vi "RT_stage_control_rev7.vi"() -> ()   [LabVIEW 2017]
uses:
  <vilib>/rvi/interface/nirviReadWriteControl/nirviReadWriteControl.xnode
  <vilib>/rvi/interface/nirviOpenFPGA/nirviOpenFPGA.xnode
  <vilib>/Platform/TimedLoop/XDataNode/XDataNode.xnode
  <vilib>/Platform/TimedLoop/XDataNode/nitl_modes.ctl
  <vilib>/Platform/TimedLoop/XDataNode/XDNodeRunTimeDep.lvlib
  <vilib>/Platform/TimedLoop/XDataNode/wakeup.ctl
  <vilib>/Platform/TimedLoop/XDataNode/timing_clust.ctl
  NiFpgaLv.dll
  <vilib>/Utility/error.llb/Error Cluster From Error Code.vi
  <vilib>/rvi/interface/Simulation/niFpgaSimulationCallBeginRW.vi
  <vilib>/rvi/errors/niLvFpgaAdjustHostInterfaceError.vi
  StageControl.ctl
  <vilib>/rvi/interface/nirviCloseFPGA/nirviCloseFPGA.xnode
  RasterControl.ctl
  <vilib>/FPGAPlugInAG/Dynamic/niLvFpga_Close_Dynamic.vi
  ForceControl.ctl
  FPGA Bitfiles/studentchallenge_FPGATarget_FPGARADCWDAC3_gNVwU-DQYMc.lvbitx
  FPGA_2R_ADC_W_DAC.vi
  <vilib>/FPGAPlugInAG/myRIO-1900/niLvFpga_Open_myRIO-1900.vi
  <vilib>/rvi/interface/common/dynamic/niFpgaDynamicAddResources.vi
panel:
  out "Force Loop":T1
  out "Force Control Late":i16
  in  "Y Manual [mm]":dbl format="%.4f"
  in  "X Manual [mm]":dbl format="%.4f"
  in  "Zero Cap":bool
  in  "Zero Y":bool
  in  "Zero X":bool
  in  "Des Force [N]":dbl=0.3 format="%.3f"
  in  "Return Speed":dbl=5.0 format="%#_13g"
  in  "Step Size [mm]":dbl=0.02 format="%.3f"
  in  "Width [mm]":dbl=3.0 format="%.3f"
  in  "Velocity [mm/s]":dbl=0.1 format="%.3f"
  in  "Stroke [mm]":dbl=3.0 format="%.3f"
  out "Current [A]":dbl=-0.00198361231060317 format="%.4f"
  out "Cap Probe [mm]":dbl=0.43435006179715263 format="%.4f"
  out "X Position [mm]":dbl format="%.4f"
  out "Y Position [mm]":dbl=0.0003125 format="%.4f"
  out "Stage Motion Late":i16
  in  "Start":bool
  in  "Operation":T2=enum."Raster"
  out "Raster Loop":T3
  out "Outer Loop":T2
  in  "stop":bool
  out "settle start":u32
  out "stroke finished":bool=TRUE
  out "ToolDownStart":bool
  out "Tool Up Finished":bool
  out "Tool Down Finished":bool
  out "FPGA Ref":refnum<k20>
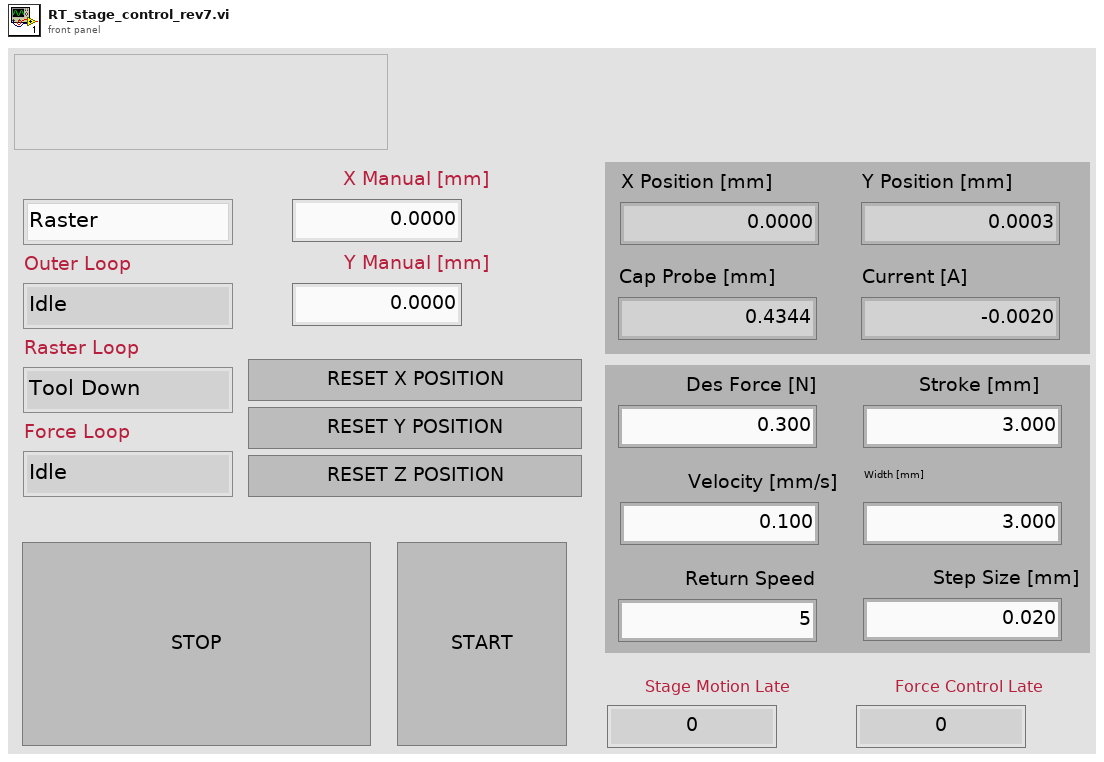
[diagram p1: front panel]
types:
  T1 = typedef "ForceControl.ctl" = enum16{"Idle", "Tool Down", "Force Control", "Tool Up"}
  T2 = typedef "StageControl.ctl" = enum16{"Idle", "Raster", "Home X", "Home Y"}
  T3 = typedef "RasterControl.ctl" = enum16{"Tool Down", "Stroke", "Tool Up", "Return & Step", "Settle", "Return to Zero"}
  T4 = cluster{"Encoder A":i32, "Encoder B":i32, "X Desired [mm]":dbl, "X Position [mm]":dbl, "Y Desired [mm]":dbl, "Y Position [mm]":dbl}
  T5 = typedef "XDNodeRunTimeDep.lvlib/timing_clust.ctl" = cluster{"Expected End [f-1]":u64, "Actual End [f-1]":u64, "Finished Late? [f-1]":bool, "Expected End [i-1]":u64, "Actual End [i-1]":u64, "Finished Late? [i-1]":bool, "Expected Start [i]":u64, "Actual Start [i]":u64, "Expected Start [f]":u64, "Actual Start [f]":u64, "Source Name":string, "Structure Name":string, "Period":i64, "Deadline":i64, "Offset":i64, "Start":i64, "Priority":i32, "Timeout":i32, "Mode":T6, "Wakeup Reason":T7, "Error":errorcluster, "Source Type":string, "Secondary Source Type":string, "Global End Time":u64, "Global Start Time":u64, "Frame Duration":u64, "Iteration Duration":u64, "Assigned CPU":i32, "I/O Scan Engine Mode":u32}
  T6 = typedef "XDNodeRunTimeDep.lvlib/nitl_modes.ctl" = enum32{"No Change", "Process missed periods, maintain original phase", "Discard missed periods, maintain original phase", "Process missed periods, ignore original phase", "Discard missed periods, ignore original phase"}
  T7 = typedef "XDNodeRunTimeDep.lvlib/wakeup.ctl" = enum32{"Normal", "Aborted", "Asynchronous wakeup", "Timing source error", "Timed loop error", "Timeout"}
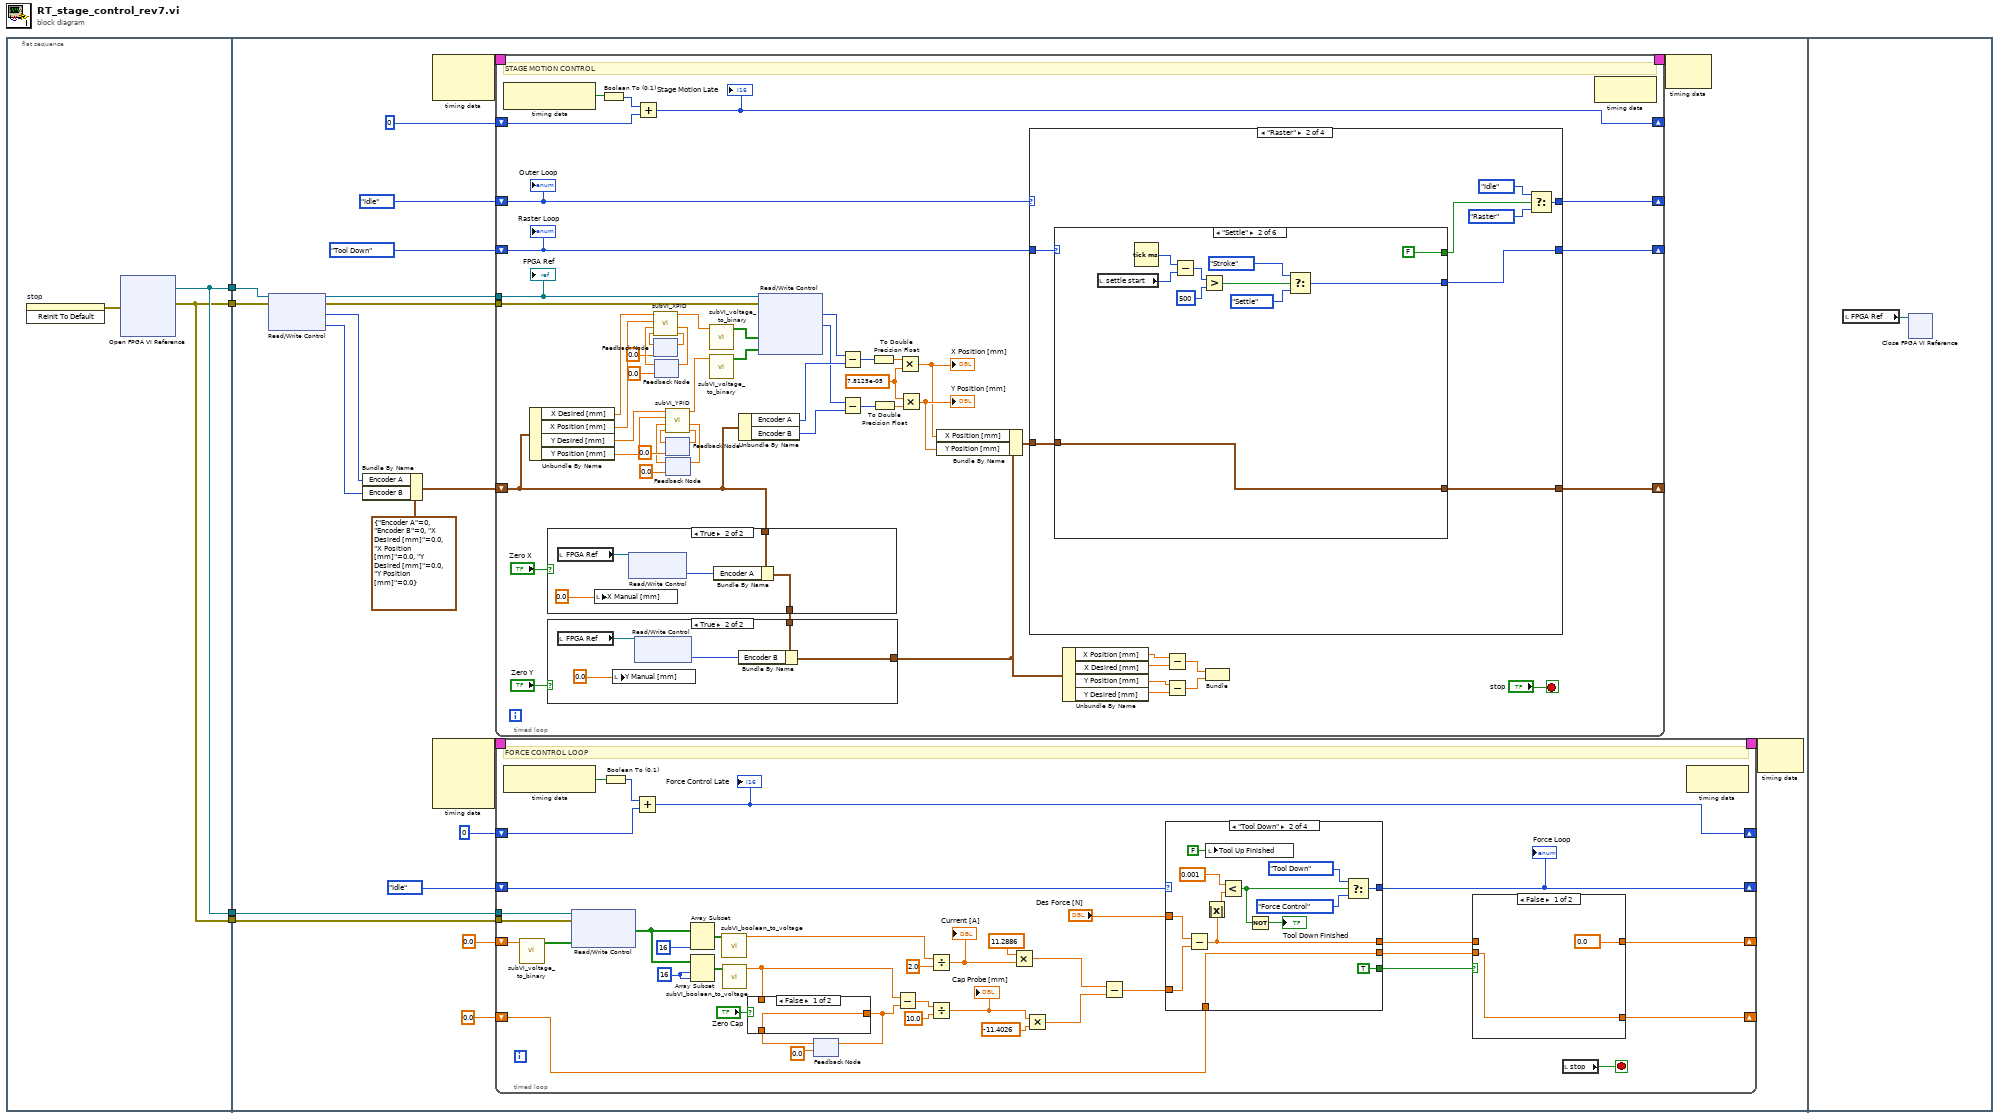
[diagram p0: block diagram]
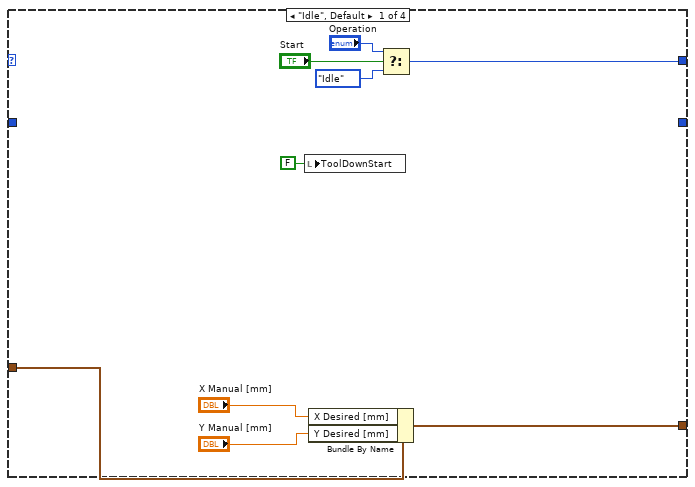
[diagram p2: hidden frame]
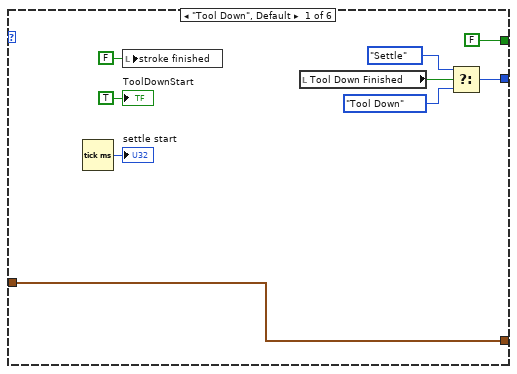
[diagram p3: hidden frame]
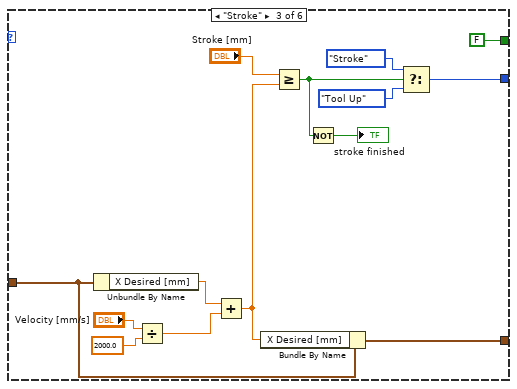
[diagram p4: hidden frame]
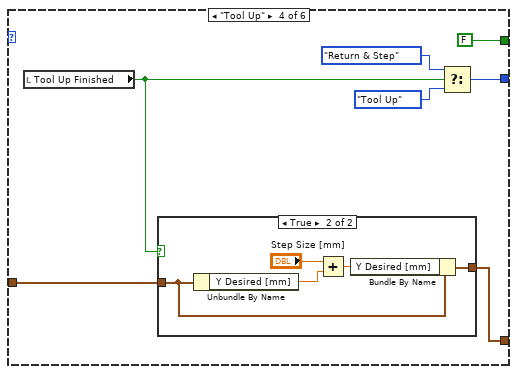
[diagram p5: hidden frame]
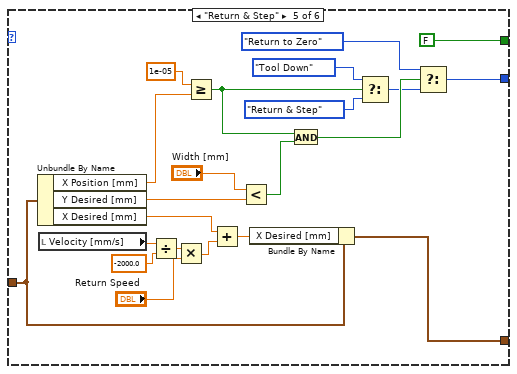
[diagram p7: hidden frame]
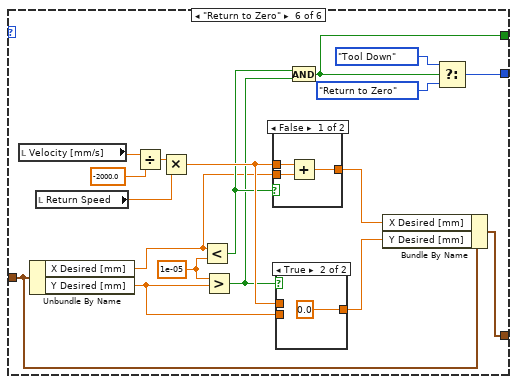
[diagram p8: hidden frame]
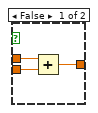
[diagram p9: hidden frame]
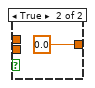
[diagram p10: hidden frame]
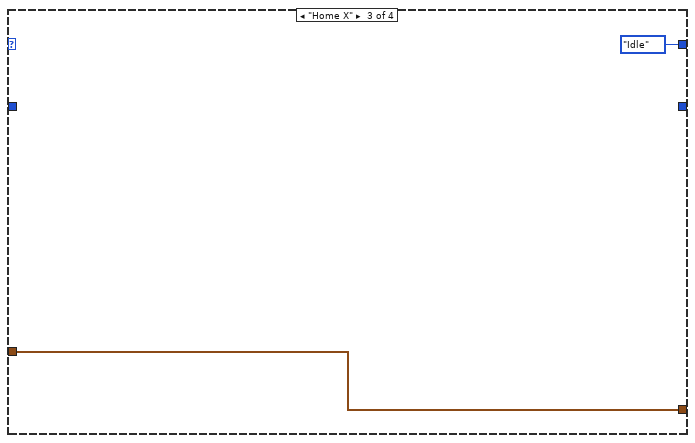
[diagram p11: hidden frame]
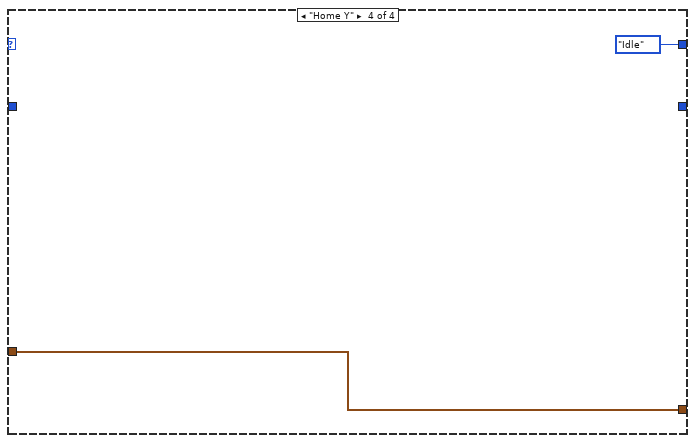
[diagram p12: hidden frame]
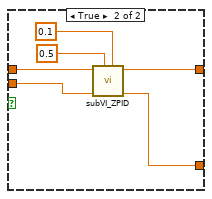
[diagram p15: hidden frame]
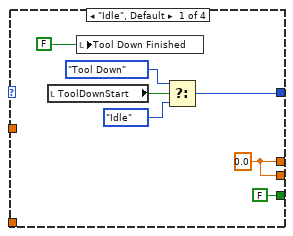
[diagram p17: hidden frame]
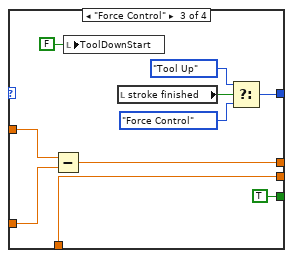
[diagram p18: hidden frame]
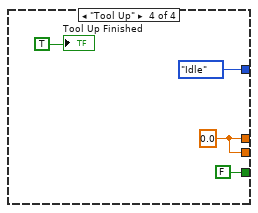
[diagram p19: hidden frame]
diagram:
  n1 = flat-sequence {
    tunnel: [w5] -> w4
    tunnel: [w6] -> w3
    tunnel: [w6] -> w2
    tunnel: [w5] -> w1
    tunnel: w4 -> [w19]
    tunnel: w3 -> [w17]
    tunnel: w2 -> [w16]
    tunnel: w1 -> [w15]
    frame #0 {
      n2 = invoke on="stop" class="Bool (strict)" method="Reinit To Default"() -> (error out=w7:errorcluster)  [unwired: 3 in, 2 out]
      n3 = xnode "Open FPGA VI Reference"("error in"=w7) -> ("FPGA VI Reference Out"=w6:refnum<k20>, "error out"=w5:errorcluster)  [unwired: 1 in]
    }
    frame #1 {
      n4 = xnode "Read/Write Control"("FPGA VI Reference In"=w17, "error in"=w19) -> ("FPGA VI Reference Out"=w24:refnum<k20>, "error out"=w23:errorcluster, "Encoder A"=w11:i32, "Encoder B"=w12:i32)
      n5 = Bundle By Name(cluster=T4 {"Encoder A"=0, "Encoder B"=0, "X Desired [mm]"=0.0, "X Position [mm]"=0.0, "Y Desired [mm]"=0.0, "Y Position [mm]"=0.0}, "Encoder A"=w11, "Encoder B"=w12) -> (w13:T4)
      n6 = node-c288() -> (w28:T5)  [unwired: 2 in]
      n7 = node-c288() -> (w26:T5)  [unwired: 4 in]
      n8 = timed-loop {
        timing: w28 -> [_]
        timing-out: [_] -> w27
        tunnel: w24 -> [w66]
        tunnel: w23 -> [w82]
        shift-right: [w76] -> _
        shift-left: StageControl."Idle" ("Enum 2") -> [w75]
        shift-right: [w73] -> _
        shift-left: RasterControl."Tool Down" -> [w74]
        shift-right: [w67] -> _
        shift-left: i16 0 -> [w68]
        shift-right: [w48] -> _
        shift-left: w13 -> [w43]
        stop <- "stop" stop-if-true
        w77 = 7.8125e-05 ("y")
        # "STAGE MOTION CONTROL"
        n9 = node-c288() -> (w70:bool)  [unwired: 1 in]
        n10 = Unbundle By Name(w43) -> ("X Desired [mm]"=w47:dbl, "X Position [mm]"=w46:dbl, "Y Desired [mm]"=w45:dbl, "Y Position [mm]"=w44:dbl)
        n11 = case shown="True" "Zero X" {
          tunnel: [w208 w210] -> w49
          tunnel: w43 -> [w208 w209]
          frame False {
          }
          frame True {
            n12 = local read "FPGA Ref"() -> (w212:refnum<k20>)
            n13 = local write "X Manual [mm]"(0.0 ("X Relative Position [mm]")) -> ()
            n14 = xnode "Read/Write Control"("FPGA VI Reference In"=w212) -> ("Encoder A"=w211:i32)  [unwired: 1 in, 2 out]
            n15 = Bundle By Name(cluster=w209, "Encoder A"=w211) -> (w210:T4)
          }
        }
        n16 = case shown="True" "Zero Y" {
          tunnel: w49 -> [w202 w206]
          tunnel: [w202 w203] -> w29
          frame False {
          }
          frame True {
            n17 = local read "FPGA Ref"() -> (w207:refnum<k20>)
            n18 = local write "Y Manual [mm]"(0.0 ("Y Relative Position [mm]")) -> ()
            n19 = xnode "Read/Write Control"("FPGA VI Reference In"=w207) -> ("Encoder B"=w205:i32)  [unwired: 1 in, 2 out]
            n20 = Bundle By Name(cluster=w206, "Encoder B"=w205) -> (w203:T4)
          }
        }
        n21 = Boolean To (0,1)(Boolean=w70) -> (0, 1=w69:i16)
        n22 = Add(x=w69, y=w68) -> (x+y=w67:i16)
        "Stage Motion Late" <- w67
        n23 = feedback #1(0.0 ("Cumulative Error Out")) -> (w61:dbl)
        n24 = feedback #2(0.0 ("Error")) -> (w60:dbl)
        n25 = call "subVI_XPID.vi"("Cumulative Error In"=w61, "Previous Error"=w60, "Encoder Position [mm]"=w46, "Desired Position [mm]"=w47) -> ("Cumulative Error Out"=w63:dbl, "Error"=w62:dbl, "Control Signal [V]"=w51:dbl)  [unwired: 5 in]
        n26 = feedback-in #1(w63) -> ()
        n27 = feedback-in #2(w62) -> ()
        n28 = feedback #3(0.0 ("Cumulative Error Out")) -> (w54:dbl)
        n29 = feedback #4(0.0 ("Error")) -> (w55:dbl)
        n30 = call "subVI_YPID.vi"("Cumulative Error In"=w54, "Previous Error"=w55, "Encoder Position [mm]"=w44, "Desired Position [mm]"=w45) -> ("Cumulative Error Out"=w52:dbl, "Error"=w53:dbl, "Control Signal [V]"=w50:dbl)  [unwired: 5 in]
        n31 = feedback-in #3(w52) -> ()
        n32 = feedback-in #4(w53) -> ()
        n33 = call "subVI_voltage_to_binary.vi"("voltage"=w51) -> ("binary"=w65:bool[])  [unwired: 10 in]
        n34 = call "subVI_voltage_to_binary.vi"("voltage"=w50) -> ("binary"=w64:bool[])  [unwired: 10 in]
        n35 = Unbundle By Name(w43) -> ("Encoder A"=w42:i32, "Encoder B"=w41:i32)
        n36 = xnode "Read/Write Control"("FPGA VI Reference In"=w66, "error in"=w82, "DAC 1 write"=w65, "DAC 2 write"=w64) -> ("Encoder A"=w40:i32, "Encoder B"=w39:i32)  [unwired: 2 out]
        n37 = Subtract(x=w40, y=w42) -> (x-y=w80:i32)
        n38 = Subtract(x=w39, y=w41) -> (x-y=w79:i32)
        n39 = To Double Precision Float(number=w80) -> (double precision float=w81:dbl)
        n40 = To Double Precision Float(number=w79) -> (double precision float=w78:dbl)
        n41 = Multiply(x=w81, y=w77) -> (x*y=w36:dbl)
        "X Position [mm]" <- w36
        n42 = Multiply(x=w77, y=w78) -> (x*y=w37:dbl)
        "Y Position [mm]" <- w37
        n43 = Bundle By Name(cluster=w29, "X Position [mm]"=w36, "Y Position [mm]"=w37) -> (w38:T4)
        n44 = case shown="\"Raster\"" w75 {
          tunnel: [w95 w102 StageControl."Idle" ("Enum 2") StageControl."Idle" ("Enum 2")] -> w76
          tunnel: w74 -> [_ w103 _ _]
          tunnel: [_ w98 _ _] -> w73
          tunnel: w38 -> [w87 w97 w198 w200]
          tunnel: [w88 w96 w198 w200] -> w48
          frame "Idle", Default {
            n45 = local write "ToolDownStart"(FALSE ("ToolDownStart")) -> ()
            n46 = Bundle By Name(cluster=w87, "X Desired [mm]"="X Manual [mm]", "Y Desired [mm]"="Y Manual [mm]") -> (w88:T4)
            n47 = Select(t="Operation", s="Start", f=StageControl."Idle" ("Enum 2")) -> (s? t:f=w95:T2)
          }
          frame "Raster" {
            n48 = case shown="\"Settle\"" w103 {
              tunnel: [FALSE FALSE FALSE FALSE FALSE w184] -> w99
              tunnel: [w111 w121 w133 w138 w154 w186] -> w98
              tunnel: [w105 w113 w130 w141 w158 w177] -> w96
              tunnel: w97 -> [w105 w113 w127 w137 w150 w174]
              frame "Tool Down", Default {
                n49 = Tick Count (ms)() -> (millisecond timer value=→"settle start":u32)
                n50 = local write "stroke finished"(FALSE ("stroke finished")) -> ()
                n51 = local read "Tool Down Finished"() -> (w108:bool)
                n52 = Select(t=RasterControl."Settle", s=w108, f=RasterControl."Tool Down") -> (s? t:f=w111:T3)
                "ToolDownStart" <- TRUE
              }
              frame "Settle" {
                n53 = local read "settle start"() -> (w114:u32)
                n54 = Tick Count (ms)() -> (millisecond timer value=w119:u32)
                n55 = Subtract(x=w119, y=w114) -> (x-y=w118:u32)
                n56 = Greater?(x=w118, y=u32 500) -> (0:w115:bool)
                n57 = Select(t=RasterControl."Stroke", s=w115, f=RasterControl."Settle") -> (s? t:f=w121:T3)
              }
              frame "Stroke" {
                n58 = Unbundle By Name(w127) -> ("X Desired [mm]"=w126:dbl)
                n59 = Divide(x="Velocity [mm/s]", y=2000.0) -> (x/y=w128:dbl)
                n60 = Add(x=w126, y=w128) -> (x+y=w125:dbl)
                n61 = Bundle By Name(cluster=w127, "X Desired [mm]"=w125) -> (w130:T4)
                n62 = Greater Or Equal?(x="Stroke [mm]", y=w125) -> (x >= y?=w124:bool)
                n63 = Not(x=w124) -> (.not. x?=→"stroke finished":bool)
                n64 = Select(t=RasterControl."Stroke", s=w124, f=RasterControl."Tool Up") -> (s? t:f=w133:T3)
              }
              frame "Tool Up" {
                n65 = local read "Tool Up Finished"() -> (w140:bool)
                n66 = case shown="True" w140 {
                  tunnel: [w144 w148] -> w141
                  tunnel: w137 -> [w144 w145]
                  frame False {
                  }
                  frame True {
                    n67 = Unbundle By Name(w145) -> ("Y Desired [mm]"=w146:dbl)
                    n68 = Add(x="Step Size [mm]", y=w146) -> (x+y=w149:dbl)
                    n69 = Bundle By Name(cluster=w145, "Y Desired [mm]"=w149) -> (w148:T4)
                  }
                }
                n70 = Select(t=RasterControl."Return & Step", s=w140, f=RasterControl."Tool Up") -> (s? t:f=w138:T3)
              }
              frame "Return & Step" {
                n71 = Unbundle By Name(w150) -> ("X Position [mm]"=w152:dbl, "Y Desired [mm]"=w151:dbl, "X Desired [mm]"=w153:dbl)
                n72 = local read "Velocity [mm/s]"() -> (w169:dbl)
                n73 = Divide(x=w169, y=-2000.0) -> (x/y=w167:dbl)
                n74 = Multiply(x=w167, y="Return Speed") -> (x*y=w159:dbl)
                n75 = Greater Or Equal?(x=1e-05 ("y"), y=w152) -> (x >= y?=w161:bool)
                n76 = Add(x=w153, y=w159) -> (x+y=w160:dbl)
                n77 = Less?(x="Width [mm]", y=w151) -> (x < y?=w155:bool)
                n78 = Bundle By Name(cluster=w150, "X Desired [mm]"=w160) -> (w158:T4)
                n79 = And(x=w161, y=w155) -> (x .and. y?=w164:bool)
                n80 = Select(t=RasterControl."Tool Down", s=w161, f=RasterControl."Return & Step") -> (s? t:f=w163:T3)
                n81 = Select(t=RasterControl."Return to Zero", s=w164, f=w163) -> (s? t:f=w154:T3)
              }
              frame "Return to Zero" {
                w181 = 1e-05 ("y")
                n82 = local read "Velocity [mm/s]"() -> (w189:dbl)
                n83 = Unbundle By Name(w174) -> ("X Desired [mm]"=w173:dbl, "Y Desired [mm]"=w172:dbl)
                n84 = local read "Return Speed"() -> (w182:dbl)
                n85 = Divide(x=w189, y=-2000.0) -> (x/y=w187:dbl)
                n86 = Multiply(x=w187, y=w182) -> (x*y=w180:dbl)
                n87 = Less?(x=w173, y=w181) -> (x < y?=w176:bool)
                n88 = Greater?(x=w181, y=w172) -> (0:w175:bool)
                n89 = case shown="False" w176 {
                  tunnel: w180 -> [w196 _]
                  tunnel: [w195 0.0] -> w179
                  tunnel: w173 -> [w194 _]
                  frame False {
                    n90 = Add(x=w196, y=w194) -> (x+y=w195:dbl)
                  }
                  frame True {
                  }
                }
                n91 = case shown="True" w175 {
                  tunnel: w180 -> [w192 _]
                  tunnel: [w191 0.0] -> w178
                  tunnel: w172 -> [w190 _]
                  frame False {
                    n92 = Add(x=w192, y=w190) -> (x+y=w191:dbl)
                  }
                  frame True {
                  }
                }
                n93 = And(x=w176, y=w175) -> (x .and. y?=w184:bool)
                n94 = Bundle By Name(cluster=w174, "X Desired [mm]"=w179, "Y Desired [mm]"=w178) -> (w177:T4)
                n95 = Select(t=RasterControl."Tool Down", s=w184, f=RasterControl."Return to Zero") -> (s? t:f=w186:T3)
              }
            }
            n96 = Select(t=StageControl."Idle" ("Enum 2"), s=w99, f=StageControl."Raster" ("Enum 2")) -> (s? t:f=w102:T2)
          }
          frame "Home X" {
          }
          frame "Home Y" {
          }
        }
        n97 = Unbundle By Name(w29) -> ("X Position [mm]"=w32:dbl, "X Desired [mm]"=w33:dbl, "Y Position [mm]"=w34:dbl, "Y Desired [mm]"=w35:dbl)
        n98 = Subtract(x=w32, y=w33) -> (x-y=w31:dbl)
        n99 = Subtract(x=w34, y=w35) -> (x-y=w30:dbl)
        n100 = Bundle(w31, w30) -> ()  [unwired: 1 in, 1 out]
        n101 = node-c288() -> ()  [unwired: 1 in, 1 out]
        "Outer Loop" <- w75
        "Raster Loop" <- w74
        "FPGA Ref" <- w66
      }
      n102 = timed-loop {
        timing: w26 -> [_]
        timing-out: [_] -> w25
        shift-right: [w215] -> _
        shift-left: ForceControl."Idle" -> [w244]
        tunnel: w16 -> [w234]
        tunnel: w15 -> [w233]
        shift-right: [w216] -> _
        shift-left: 0.0 -> [w230]
        shift-right: [w224] -> _
        shift-left: 0.0 ("Cumulative Error Out") -> [w222]
        shift-right: [w218] -> _
        shift-left: i16 0 -> [w221]
        stop <- w253 stop-if-true
        w251 = 16 ("length")
        # "FORCE CONTROL LOOP"
        n103 = node-c288() -> (w220:bool)  [unwired: 1 in]
        n104 = call "subVI_voltage_to_binary.vi"("voltage"=w230) -> ("binary"=w231:bool[])  [unwired: 10 in]
        n105 = xnode "Read/Write Control"("FPGA VI Reference In"=w234, "error in"=w233, "DAC 3 write"=w231) -> ("ADC Read"=w243:bool[])  [unwired: 2 out]
        n106 = Boolean To (0,1)(Boolean=w220) -> (0, 1=w219:i16)
        n107 = Add(x=w219, y=w221) -> (x+y=w218:i16)
        "Force Control Late" <- w218
        n108 = Array Subset(array=w243, length=16) -> (w252:bool[])  [unwired: 1 in]
        n109 = Array Subset(array=w243, index=w251, length=w251) -> (w250:bool[])
        n110 = call "subVI_boolean_to_voltage.vi"("ADC read"=w252) -> ("V"=w225:dbl)  [unwired: 10 in]
        n111 = call "subVI_boolean_to_voltage.vi"("ADC read"=w250) -> ("V"=w237:dbl)  [unwired: 10 in]
        n112 = feedback #5(0.0) -> (w236:dbl)
        n113 = case shown="False" "Zero Cap" {
          tunnel: [w262 w263] -> w232
          tunnel: w236 -> [w262 _]
          tunnel: w237 -> [_ w263]
          frame False {
          }
          frame True {
          }
        }
        n114 = feedback-in #5(w232) -> ()
        n115 = Subtract(x=w237, y=w232) -> (x-y=w240:dbl)
        n116 = Divide(x=w225, y=2.0) -> (x/y=w245:dbl)
        "Current [A]" <- w245
        n117 = Divide(x=w240, y=10.0) -> (x/y=w235:dbl)
        "Cap Probe [mm]" <- w235
        n118 = Multiply(x=11.2886 ("BL"), y=w245) -> (x*y=w242:dbl)
        n119 = Multiply(x=w235, y=-11.4026 ("Stiffness [N/m]")) -> (x*y=w241:dbl)
        n120 = Subtract(x=w242, y=w241) -> (x-y=w226:dbl)
        n121 = case shown="\"Tool Down\"" w244 {
          tunnel: [w267 w281 w293 ForceControl."Idle"] -> w215
          tunnel: "Des Force [N]" -> [_ w279 w287 _]
          tunnel: w226 -> [_ w278 w286 _]
          tunnel: [w264 w275 w288 w294] -> w228
          tunnel: [FALSE TRUE TRUE FALSE] -> w217
          tunnel: [w264 w271 w284 w294] -> w223
          tunnel: w222 -> [_ w271 w284 _]
          frame "Idle", Default {
            w264 = 0.0
            n122 = local read "ToolDownStart"() -> (w268:bool)
            n123 = local write "Tool Down Finished"(FALSE ("Tool Down Finished")) -> ()
            n124 = Select(t=ForceControl."Tool Down", s=w268, f=ForceControl."Idle") -> (s? t:f=w267:T1)
          }
          frame "Tool Down" {
            n125 = Subtract(x=w279, y=w278) -> (x-y=w275:dbl)
            n126 = Absolute Value(x=w275) -> (abs(x)=w276:dbl)
            n127 = local write "Tool Up Finished"(FALSE ("Tool Up Finished")) -> ()
            n128 = Less?(x=0.001 ("error threshold"), y=w276) -> (x < y?=w273:bool)
            n129 = Not(x=w273) -> (.not. x?=→"Tool Down Finished":bool)
            n130 = Select(t=ForceControl."Tool Down", s=w273, f=ForceControl."Force Control") -> (s? t:f=w281:T1)
          }
          frame "Force Control" {
            n131 = Subtract(x=w287, y=w286) -> (x-y=w288:dbl)
            n132 = local write "ToolDownStart"(FALSE ("ToolDownStart")) -> ()
            n133 = local read "stroke finished"() -> (w292:bool)
            n134 = Select(t=ForceControl."Tool Up", s=w292, f=ForceControl."Force Control") -> (s? t:f=w293:T1)
          }
          frame "Tool Up" {
            w294 = 0.0
            "Tool Up Finished" <- TRUE ("Tool Up Finished")
          }
        }
        "Force Loop" <- w215
        n135 = case shown="False" w217 {
          tunnel: w228 -> [_ w261]
          tunnel: [0.0 ("Z Manual") w260] -> w216
          tunnel: [w254 w257] -> w224
          tunnel: w223 -> [w254 w256]
          frame False {
          }
          frame True {
            n136 = call "subVI_ZPID.vi"("I"=0.1, "P"=0.5, "Cumulative Error In"=w256, "Error In"=w261) -> ("Cumulative Error Out"=w257:dbl, "Control Signal [V]"=w260:dbl)  [unwired: 6 in]
          }
        }
        n137 = local read "stop"() -> (w253:bool)
        n138 = node-c288() -> ()  [unwired: 1 in, 1 out]
      }
      n139 = node-c288(w27) -> ()  [unwired: 1 out]
      n140 = node-c288(w25) -> ()  [unwired: 1 out]
    }
    frame #2 {
      n141 = local read "FPGA Ref"() -> (w304:refnum<k20>)
      n142 = xnode "Close FPGA VI Reference"("FPGA VI Reference In"=w304) -> ()  [unwired: 1 in, 1 out]
    }
  }
